vi "Test Panther Dashboard API.vi"() -> ()   [LabVIEW 2023]
doc: "Panther Dashboard API Tester.\n\n<b>Note:</b> This VI was modified by the <b>Validate DQMH Module</b> tool to remove code to stop the main loop on error, and instead display the most recent error on the tester front panel."
uses:
  DQMH Tools Menu--enum.ctl
  <vilib>/Utility/error.llb/DialogType.ctl
  Panther Dashboard.lvlib
panel:
  in  "Save Module Spec":bool
  out "last error":errorcluster
  in  "Project Description":string
  in  "Save Project Documentation":bool
  in  "Open Documentation":bool
  in  "VI Description":string
  in  "Save VI Description":bool
  in  "Library Description":string
  in  "Save Library Description":bool
  in  "New ID":i32=-1 min=-1 max=1000 step=1 format="Module ID %d"
  in  "Update Module ID":bool
  out "Event Connector Pane":picture
  in  "About":bool=TRUE
  in  "Theme":bool=TRUE
  in  "Generate Project Documentation":bool
  in  "Scripting Tool":T1
  in  "Launch DQMH Scripting Tools":bool
  in  "Targets":string(combo)
  in  "Projects":string(combo)
  in  "Expand or Close":bool
  in  "Include Dependencies":bool
  in  "Scan DQMH Modules":bool
  in  "Show Diagram on Init":bool
  in  "Show Block Diagram":bool
  in  "Stop Module":bool
  in  "Start Module":bool
  in  "Hide Module Panel":bool
  in  "Show Module Panel":bool
  out "Status":string
  out "Module Running?":bool
  # "This VI tests the API for the Module."
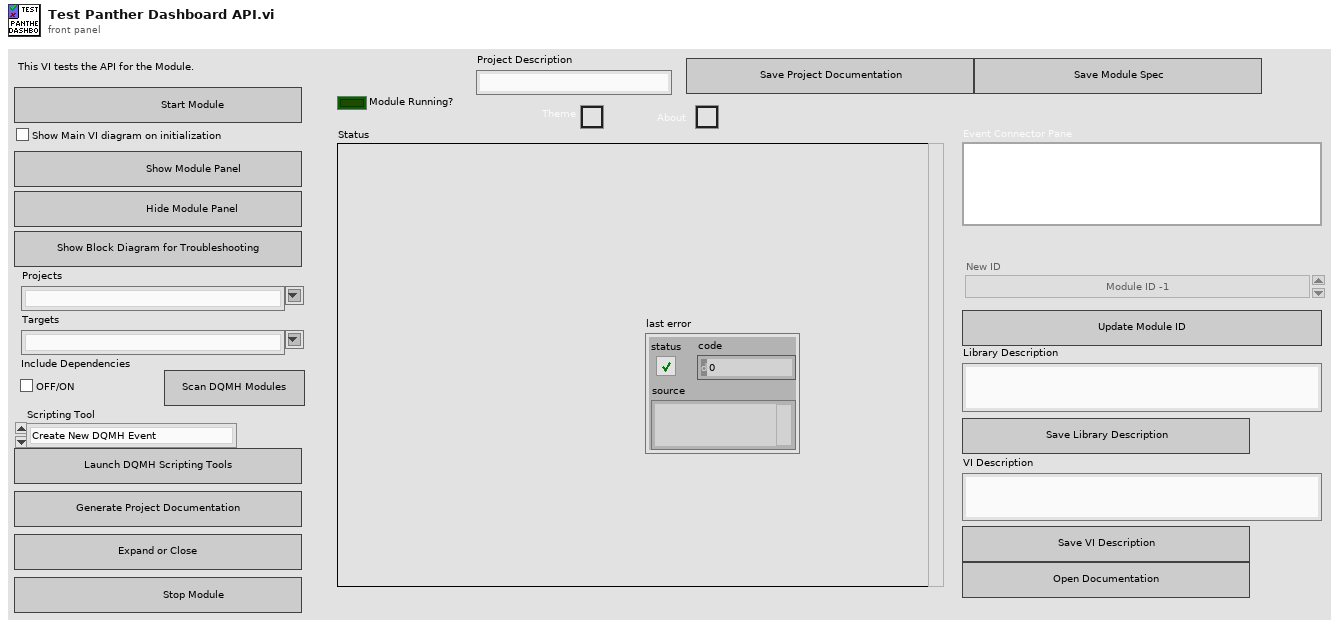
[diagram p1: front panel]
types:
  T1 = typedef "Panther Dashboard.lvlib/DQMH Tools Menu--enum.ctl" = enum16{"Create New DQMH Event", "Remove DQMH Event", "Convert DQMH Event", "Rename DQMH Event", "Add New DQMH Module", "Create RT Tester", "Rename DQMH Module", "Validate DQMH Module", "Create DQMH Module Template", "New DQMH  Unit Test", "Add Helper Loop to DQMH Module"}
  T2 = typedef "Panther Dashboard.lvlib/Broadcast Events--cluster.ctl" = cluster{"Module Did Init":refnum<user-event>, "Status Updated":refnum<user-event>, "Error Reported":refnum<user-event>, "Module Did Stop":refnum<user-event>, "Update Module Execution Status":refnum<user-event>, "References Updated":refnum<user-event>, "Projects Updated":refnum<user-event>, "Targets Updated":refnum<user-event>, "Progress updated":refnum<user-event>, "Scale Updated":refnum<user-event>, "Connector Pane Updated":refnum<user-event>, "Documentation Updated":refnum<user-event>, "Module Type Updated":refnum<user-event>, "Theme Updated":refnum<user-event>, "Project Description Updated":refnum<user-event>}
  T3 = typedef "DialogType.ctl" = u16
  T4 = typedef "Panther Dashboard.lvlib/Module type--enum.ctl" = enum16{"Singleton", "Cloneable"}
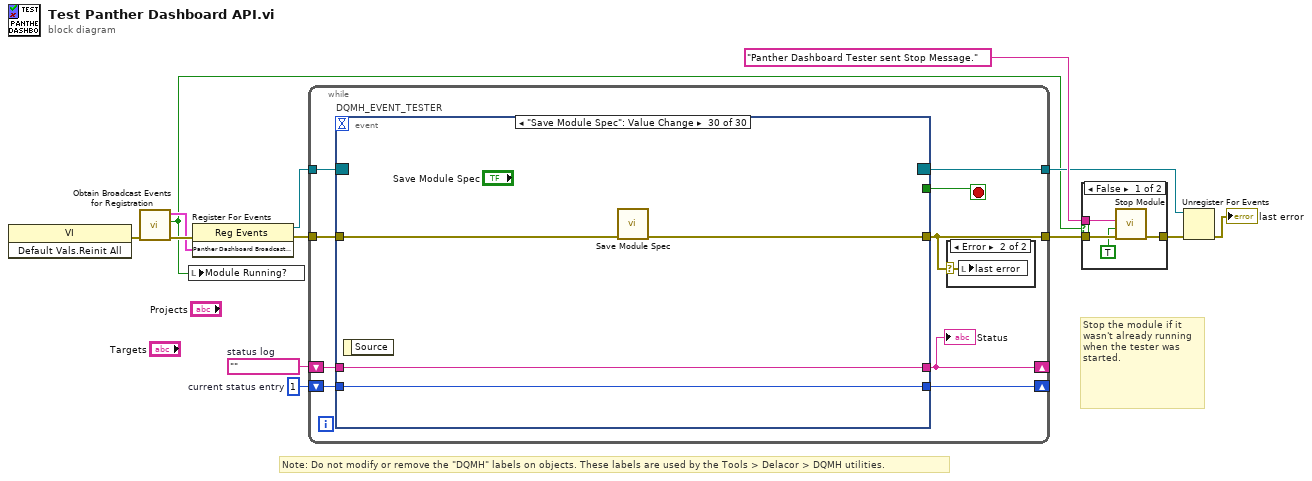
[diagram p0: block diagram]
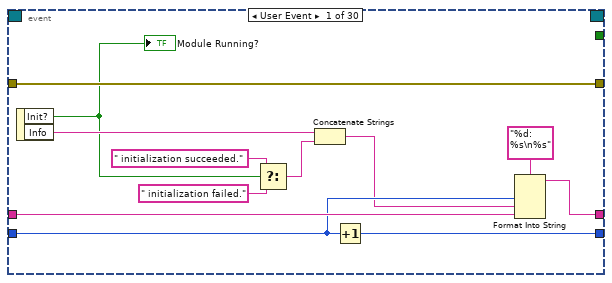
[diagram p4: hidden frame]
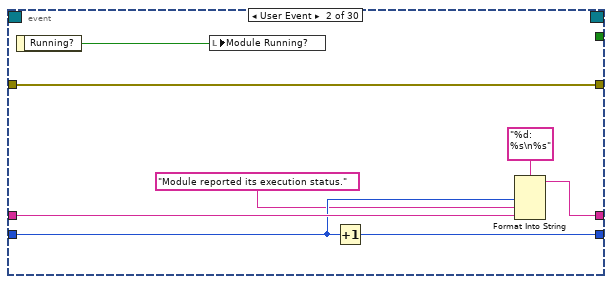
[diagram p5: hidden frame]
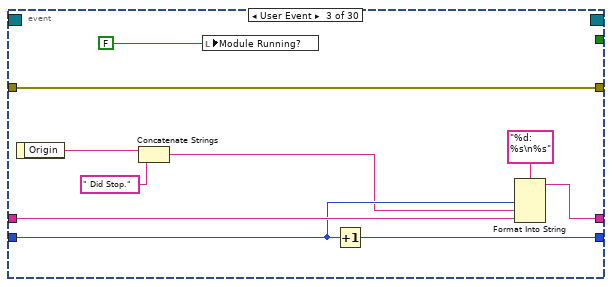
[diagram p6: hidden frame]
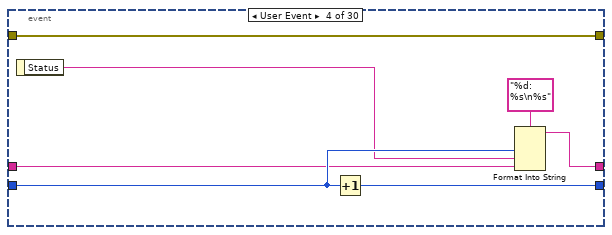
[diagram p7: hidden frame]
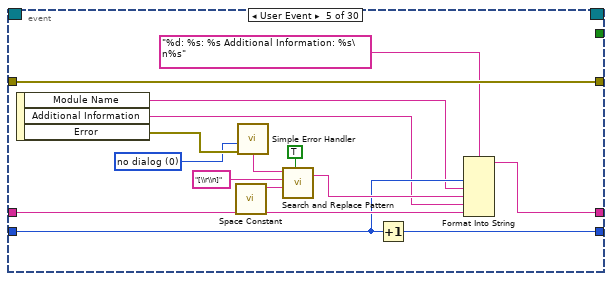
[diagram p8: hidden frame]
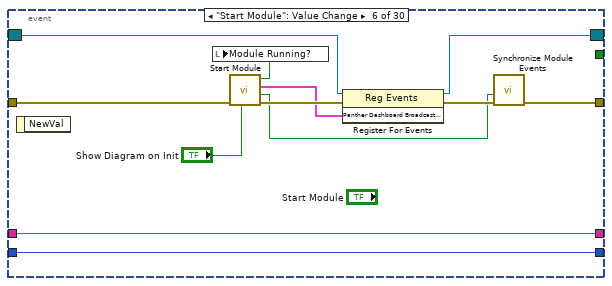
[diagram p9: hidden frame]
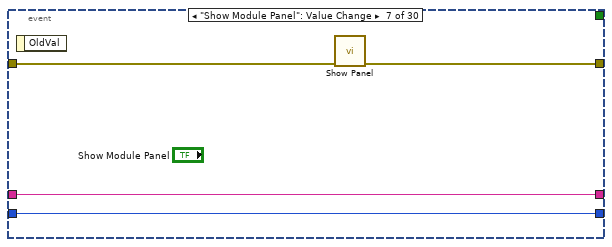
[diagram p10: hidden frame]
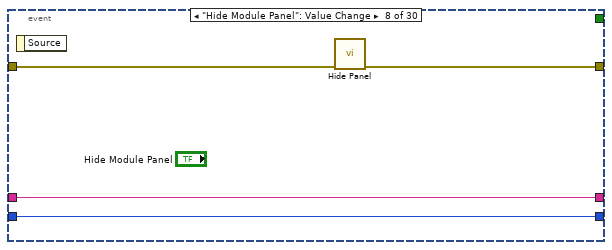
[diagram p11: hidden frame]
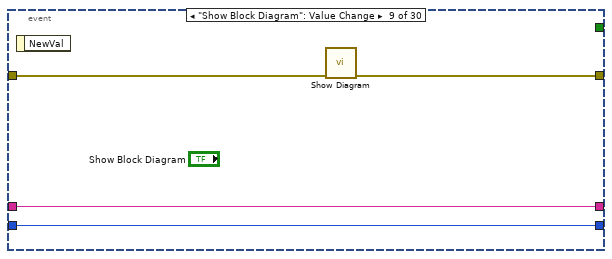
[diagram p12: hidden frame]
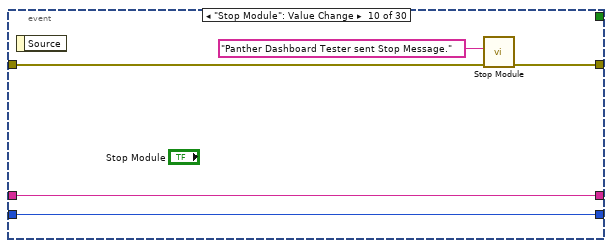
[diagram p13: hidden frame]
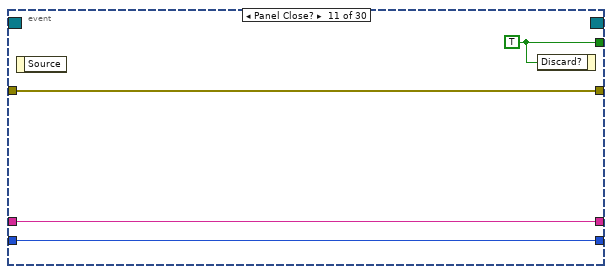
[diagram p14: hidden frame]
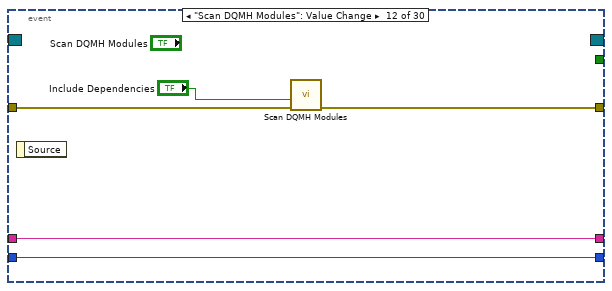
[diagram p15: hidden frame]
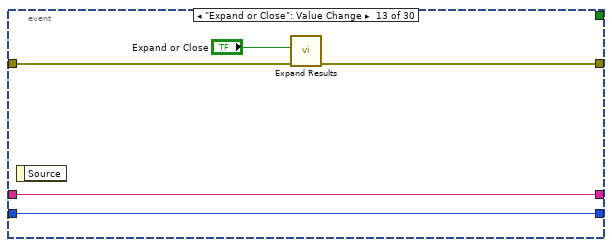
[diagram p16: hidden frame]
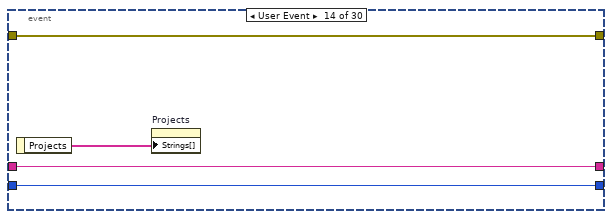
[diagram p17: hidden frame]
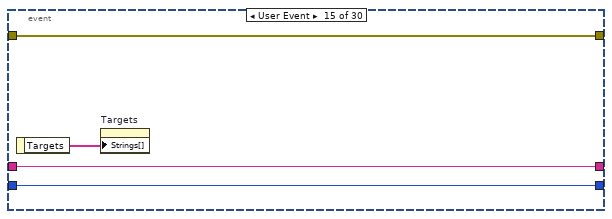
[diagram p18: hidden frame]
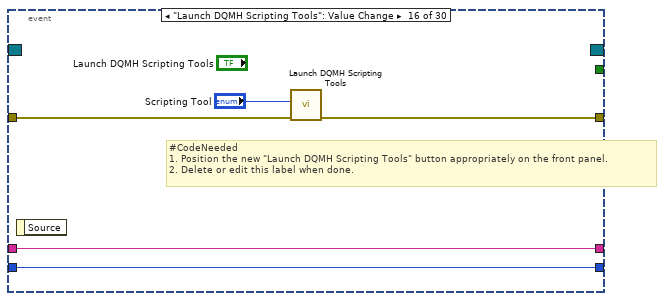
[diagram p19: hidden frame]
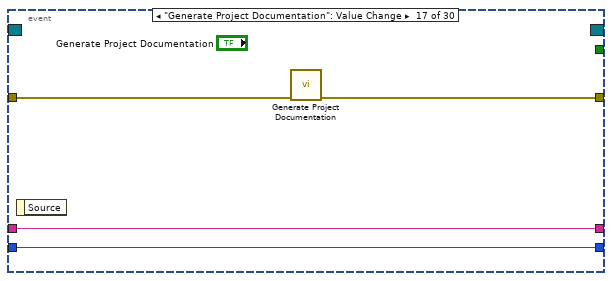
[diagram p20: hidden frame]
diagram:
  w5 = 1  # current status entry
  w6 = ""  # status log
  # "Stop the module if it wasn't already running when the tester was started."
  # "Note: Do not modify or remove the \"DQMH\" labels on objects. These labels are used by the Tools > Delacor > DQMH utilities."
  n1 = invoke class="VI" method="Default Vals.Reinit All"() -> (error out=w11:errorcluster)  [unwired: 3 in, 2 out]
  n2 = call "Obtain Broadcast Events for Registration.vi"("error in"=w11) -> ("error out"=w10:errorcluster, "Already running?"=w1:bool, "Panther Dashboard Broadcast Events"=w4:T2)  [unwired: 8 in]
  n3 = local write "Module Running?"(w1) -> ()
  n4 = register-events(error in=w10, w4) -> (reference out=w3:refnum<event-registration>, error out=w12:errorcluster)  [unwired: 1 in]
  n5 = while {
    tunnel: w3 -> [w20]
    tunnel: [w21] -> w9
    shift-right: [w16] -> _
    shift-left: w6 -> [w18]
    shift-right: [w17] -> _
    shift-left: w5 -> [w19]
    tunnel: w12 -> [w22]
    tunnel: [w15] -> w2
    stop <- w14 stop-if-true
    n6 = event "DQMH_EVENT_TESTER" shown="[29] \"Save Module Spec\": Value Change" {
      selector: w20 -> [_ _ _ _ _ w79 _ _ _ _ _ _ _ _ _ _ _ _ _ _ _ _ _ _ _ _ _ _ _ _]
      dyn-events: [_ _ _ _ _ w78 _ _ _ _ _ _ _ _ _ _ _ _ _ _ _ _ _ _ _ _ _ _ _ _] -> w15
      timeout: _ -> [_ _ _ _ _ _ _ _ _ _ _ _ _ _ _ _ _ _ _ _ _ _ _ _ _ _ _ _ _ _]
      tunnel: [_ _ _ _ _ _ _ _ _ _ w107 _ _ _ _ _ _ _ _ _ _ _ _ _ _ _ _ _ _ _] -> w14
      tunnel: [w35 w43 w53 w60 w75 w85 w91 w95 w98 w104 w108 w112 w117 w122 w126 w130 w134 w139 w143 w148 w158 w162 w172 w176 w181 w191 w194 w204 w208 w210] -> w21
      tunnel: w19 -> [w32 w40 w50 w56 w65 w82 w88 w92 w96 w101 w105 w110 w115 w120 w124 w128 w132 w137 w141 w146 w155 w160 w169 w174 w179 w188 w192 w201 w206 w211]
      tunnel: w18 -> [w33 w41 w51 w55 w66 w83 w89 w93 w97 w102 w106 w111 w116 w121 w125 w129 w133 w138 w142 w147 w157 w161 w171 w175 w180 w190 w193 w203 w207 w212]
      tunnel: [w30 w38 w48 w57 w64 w83 w89 w93 w97 w102 w106 w111 w116 w121 w125 w129 w133 w138 w142 w147 w156 w161 w170 w175 w180 w189 w193 w202 w207 w212] -> w16
      tunnel: [w31 w39 w49 w59 w63 w82 w88 w92 w96 w101 w105 w110 w115 w120 w124 w128 w132 w137 w141 w146 w154 w160 w168 w174 w179 w187 w192 w200 w206 w211] -> w17
      tunnel: w22 -> [w35 w43 w53 w60 w75 w84 w90 w94 w99 w103 w108 w113 w118 w122 w126 w131 w135 w140 w144 w148 w158 w163 w172 w177 w182 w191 w195 w204 w209 w213]
      event User Event {
        n7 = event-data() -> ("Init?"=w27:bool, "Info"=w29:string)  [unwired: 1 in]
        "Module Running?" <- w27
        n8 = Select(t=" initialization succeeded.", s=w27, f=" initialization failed.") -> (s? t:f=w24:string)
        n9 = Concatenate Strings(w29, w24) -> (w28:string)
        n10 = Increment(x=w32) -> (x+1=w31:i32)
        n11 = Format Into String(format string="%d: %s\n%s", w32, w28, w33) -> (resulting string=w30:string)  [unwired: 2 in, 1 out]
      }
      event User Event {
        n12 = event-data() -> ("Running?"=w36:bool)  [unwired: 1 in]
        n13 = local write "Module Running?"(w36) -> ()
        n14 = Increment(x=w40) -> (x+1=w39:i32)
        n15 = Format Into String(format string="%d: %s\n%s", w40, "Module reported its execution status.", w41) -> (resulting string=w38:string)  [unwired: 2 in, 1 out]
      }
      event User Event {
        n16 = event-data() -> ("Origin"=w47:string)  [unwired: 1 in]
        n17 = Concatenate Strings(w47, " Did Stop.") -> (w46:string)
        n18 = local write "Module Running?"(FALSE ("Module Did Init?")) -> ()
        n19 = Increment(x=w50) -> (x+1=w49:i32)
        n20 = Format Into String(format string="%d: %s\n%s", w50, w46, w51) -> (resulting string=w48:string)  [unwired: 2 in, 1 out]
      }
      event User Event {
        n21 = event-data() -> ("Status"=w54:string)  [unwired: 1 in]
        n22 = Increment(x=w56) -> (x+1=w59:i32)
        n23 = Format Into String(format string="%d: %s\n%s", w56, w54, w55) -> (resulting string=w57:string)  [unwired: 2 in, 1 out]
      }
      event User Event {
        w67 = T3 0 items=["no dialog", "OK message", "continue or stop message", "OK message + warnings", "continue/stop + warnings"] ("type of dialog (OK msg:1)")
        n24 = event-data() -> ("Module Name"=w62:string, "Additional Information"=w61:string, "Error"=w74:errorcluster)  [unwired: 1 in]
        n25 = call <vilib>:"Space Constant.vi"() -> ("String"=w71:string)
        n26 = call <vilib>:"Simple Error Handler.vi"("type of dialog (OK msg:1)"=w67, "error in (no error)"=w74) -> ("message"=w68:string)  [unwired: 3 in, 4 out]
        n27 = call <vilib>:"Search and Replace Pattern.vi"("string"=w68, "regular expression (\"\")"="[\\r\\n]" ("regular expression (\"\")"), "replace string (\"\")"=w71, "replace all? (F)"=TRUE ("replace all CR/LF with spaces")) -> ("result string"=w69:string)  [unwired: 1 in, 1 out]
        n28 = Increment(x=w65) -> (x+1=w63:i32)
        n29 = Format Into String(format string="%d: %s: %s Additional Information: %s\n%s", w65, w62, w69, w61, w66) -> (resulting string=w64:string)  [unwired: 2 in, 1 out]
      }
      event "Start Module": Value Change {
        n30 = event-data() -> ()  [unwired: 1 in, 1 out]
        n31 = call "Start Module.vi"("Show Main VI Diagram on Init (F)"="Show Diagram on Init", "error in"=w84) -> ("error out"=w86:errorcluster, "Wait for Event Sync?"=w81:bool, "Panther Dashboard Broadcast Events"=w80:T2, "Module Was Already Running?"=w77:bool)  [unwired: 6 in]
        n32 = local write "Module Running?"(w77) -> ()
        n33 = register-events(reference=w79, error in=w86, w80) -> (reference out=w78:refnum<event-registration>, error out=w87:errorcluster)
        n34 = call "Synchronize Module Events.vi"("error in"=w87, "Wait for Event Sync?"=w81) -> ("error out"=w85:errorcluster)  [unwired: 9 in]
      }
      event "Show Module Panel": Value Change {
        n35 = event-data() -> ()  [unwired: 1 in, 1 out]
        n36 = call "Show Panel.vi"("error in (no error)"=w90) -> ("error out"=w91:errorcluster)  [unwired: 10 in]
      }
      event "Hide Module Panel": Value Change {
        n37 = event-data() -> ()  [unwired: 1 in, 1 out]
        n38 = call "Hide Panel.vi"("error in (no error)"=w94) -> ("error out"=w95:errorcluster)  [unwired: 10 in]
      }
      event "Show Block Diagram": Value Change {
        n39 = event-data() -> ()  [unwired: 1 in, 1 out]
        n40 = call "Show Diagram.vi"("error in (no error)"=w99) -> ("error out"=w98:errorcluster)  [unwired: 10 in]
      }
      event "Stop Module": Value Change {
        n41 = event-data() -> ()  [unwired: 1 in, 1 out]
        n42 = call "Stop Module.vi"("error in"=w103, "Origin"="Panther Dashboard Tester sent Stop Message.") -> ("error out"=w104:errorcluster)  [unwired: 9 in]
      }
      event Panel Close? {
        w107 = TRUE ("Discard?")
        n43 = event-data() -> ()  [unwired: 1 in, 1 out]
        n44 = event-data("Discard?"=w107) -> ()  [unwired: 1 in, 1 out]
      }
      event "Scan DQMH Modules": Value Change {
        n45 = event-data() -> ()  [unwired: 1 in, 1 out]
        n46 = call "Scan DQMH Modules.vi"("error in"=w113, "Include Dependencies"="Include Dependencies") -> ("error out"=w112:errorcluster)  [unwired: 9 in]
      }
      event "Expand or Close": Value Change {
        n47 = event-data() -> ()  [unwired: 1 in, 1 out]
        n48 = call "Expand Results.vi"("error in"=w118, "Expand?"="Expand or Close") -> ("error out"=w117:errorcluster)  [unwired: 9 in]
      }
      event User Event {
        n49 = event-data() -> ("Projects"=w119:string[])  [unwired: 1 in]
        n50 = property on="Projects" class="CmbBox"("Strings[]"=w119) -> ()  [unwired: 2 in, 2 out]
      }
      event User Event {
        n51 = event-data() -> ("Targets"=w123:string[])  [unwired: 1 in]
        n52 = property on="Targets" class="CmbBox"("Strings[]"=w123) -> ()  [unwired: 2 in, 2 out]
      }
      event "Launch DQMH Scripting Tools": Value Change {
        # "#CodeNeeded\n1. Position the new \"Launch DQMH Scripting Tools\" button appropriately on the front panel.\n2. Delete or edit this label when done."
        n53 = event-data() -> ()  [unwired: 1 in, 1 out]
        n54 = call "Launch DQMH Scripting Tools.vi"("error in"=w131, "Scripting Tool"="Scripting Tool") -> ("error out"=w130:errorcluster)  [unwired: 9 in]
      }
      event "Generate Project Documentation": Value Change {
        n55 = event-data() -> ()  [unwired: 1 in, 1 out]
        n56 = call "Generate Project Documentation.vi"("error in"=w135) -> ("error out"=w134:errorcluster)  [unwired: 10 in]
      }
      event "Theme": Value Change {
        n57 = event-data() -> ()  [unwired: 1 in, 1 out]
        n58 = call "Set App Theme.vi"("error in"=w140, "Theme"="Theme") -> ("error out"=w139:errorcluster)  [unwired: 9 in]
      }
      event "About": Value Change {
        n59 = event-data() -> ()  [unwired: 1 in, 1 out]
        n60 = call "Show About.vi"("error in"=w144) -> ("error out"=w143:errorcluster)  [unwired: 10 in]
      }
      event User Event {
        n61 = event-data() -> ("Event Connector Pane"=→"Event Connector Pane":picture)  [unwired: 1 in]
      }
      event User Event {
        n62 = event-data() -> ("Documentation.Module Description"=w150:string, "Documentation.Event Description"=w149:string)  [unwired: 1 in]
        n63 = Format Into String(format string="Documentation Updated [  %s, %s]", w150, w149) -> (resulting string=w151:string)  [unwired: 2 in, 1 out]
        n64 = Increment(x=w155) -> (x+1=w154:i32)
        n65 = Format Into String(format string="%d: %s\n%s", w155, w151, w157) -> (resulting string=w156:string)  [unwired: 2 in, 1 out]
      }
      event "Update Module ID": Value Change {
        # "#CodeNeeded\n1. Position the new \"Update Module ID\" button appropriately on the front panel.\n2. Delete or edit this label when done."
        n66 = event-data() -> ()  [unwired: 1 in, 1 out]
        n67 = call "Update Module ID.vi"("error in"=w163, "New ID"="New ID") -> ("error out"=w162:errorcluster)  [unwired: 9 in]
      }
      event User Event {
        n68 = event-data() -> ("Module Type"=w164:T4)  [unwired: 1 in]
        n69 = Format Into String(format string="Module Type - %s", w164) -> (resulting string=w165:string)  [unwired: 2 in, 1 out]
        n70 = Increment(x=w169) -> (x+1=w168:i32)
        n71 = Format Into String(format string="%d: %s\n%s", w169, w165, w171) -> (resulting string=w170:string)  [unwired: 2 in, 1 out]
      }
      event "Save Library Description": Value Change {
        # "#CodeNeeded\n1. Position the new \"Save Library Description\" button appropriately on the front panel.\n2. Delete or edit this label when done."
        n72 = event-data() -> ()  [unwired: 1 in, 1 out]
        n73 = call "Save Library Description.vi"("error in"=w177, "Library Description"="Library Description") -> ("error out"=w176:errorcluster)  [unwired: 9 in]
      }
      event "Save VI Description": Value Change {
        n74 = event-data() -> ()  [unwired: 1 in, 1 out]
        n75 = call "Save VI Description.vi"("error in"=w182, "VI Description"="VI Description") -> ("error out"=w181:errorcluster)  [unwired: 9 in]
      }
      event User Event {
        n76 = event-data() -> ("Theme"=w183:bool)  [unwired: 1 in]
        n77 = Format Into String(format string="Theme Updated - %s", w183) -> (resulting string=w184:string)  [unwired: 2 in, 1 out]
        n78 = Increment(x=w188) -> (x+1=w187:i32)
        n79 = Format Into String(format string="%d: %s\n%s", w188, w184, w190) -> (resulting string=w189:string)  [unwired: 2 in, 1 out]
      }
      event "Open Documentation": Value Change {
        n80 = event-data() -> ()  [unwired: 1 in, 1 out]
        n81 = call "Open Documentation.vi"("error in"=w195) -> ("error out"=w194:errorcluster)  [unwired: 10 in]
      }
      event User Event {
        n82 = event-data() -> ("Project Description"=w196:string)  [unwired: 1 in]
        n83 = Format Into String(format string="Project Description: - %s", w196) -> (resulting string=w197:string)  [unwired: 2 in, 1 out]
        n84 = Increment(x=w201) -> (x+1=w200:i32)
        n85 = Format Into String(format string="%d: %s\n%s", w201, w197, w203) -> (resulting string=w202:string)  [unwired: 2 in, 1 out]
      }
      event "Save Project Documentation": Value Change {
        n86 = event-data() -> ()  [unwired: 1 in, 1 out]
        n87 = call "Save Project Documentation.vi"("error in"=w209, "Project Description"="Project Description") -> ("error out"=w208:errorcluster)  [unwired: 9 in]
      }
      event "Save Module Spec": Value Change {
        n88 = event-data() -> ()  [unwired: 1 in, 1 out]
        n89 = call "Save Module Spec.vi"("error in"=w213) -> ("error out"=w210:errorcluster)  [unwired: 10 in]
      }
    }
    "Status" <- w16
    n90 = case "DQMH_TESTER_ERROR_LOCAL" shown="Error" w21 {
      selector: w21 -> [_ w23]
      frame No Error {
      }
      frame Error {
        n91 = local write "last error"(w23) -> ()
      }
    }
  }
  n92 = case shown="False" w1 {
    tunnel: [w217 w218] -> w13
    tunnel: "Panther Dashboard Tester sent Stop Message." ("Origin") -> [w215 _]
    tunnel: w9 -> [w216 w218]
    frame False {
      n93 = call "Stop Module.vi"("error in"=w216, "Wait for Module to Stop? (F)"=TRUE ("Wait for Module to stop?"), "Origin"=w215) -> ("error out"=w217:errorcluster)  [unwired: 8 in]
    }
    frame True {
    }
  }
  n94 = Unregister For Events(event registration refnum=w2, error in=w13) -> (error out=→"last error":errorcluster)
